vi "SWLDA.vi"(5 "premove":dbl=0.5, 7 "penter":dbl=0.4, 8 "Maximum_Iteration":dbl=88.0, 10 "ERP_NonTarget":path=path "C:/Users/Jaehong/Desktop/안전복지프로젝트/LabVIEW/RSVP_offline_onine/분석데이터/전선미_RSVP_Training_Test(LDA)/2014-08-29/ERP_Parameters_of_NonTarget_prior.txt", 11 "ERP_Target":path=path "C:/Users/Jaehong/Desktop/안전복지프로젝트/LabVIEW/RSVP_offline_onine/분석데이터/전선미_RSVP_Training_Test(LDA)/2014-08-29/ERP_Parameters_of_Target_prior.txt") -> (0 "in":dbl[](array[numeric]), 3 "Weight":dbl[](array[numeric]))   [LabVIEW 2014]
uses:
  <vilib>/Analysis/baseanly.llb/Vector x A.vi
  <vilib>/Utility/file.llb/Read From Spreadsheet File (DBL).vi
  <vilib>/Analysis/Matrix/Numeric/Conversions/Array To Matrix - RA.vi
  <vilib>/Analysis/NI_AALBase.lvlib
  <vilib>/Analysis/Matrix/NI_Matrix.lvlib
panel:
  out "biase":dbl[](array[numeric])
  out "Nontarget_mean":dbl[](array[numeric])
  out "Target_mean":dbl[](array[numeric])
  out "Label":dbl[](array[numeric])
  # "Target/Non-Target of MATLAB"
  # "var_argin part of MATLAB"
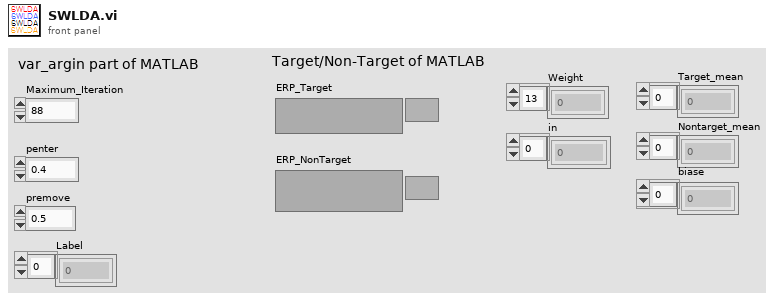
[diagram p1: front panel]
types:
  T1 = typedef "NI_Matrix.lvlib/RealMatrix.ctl" = dbl[][]
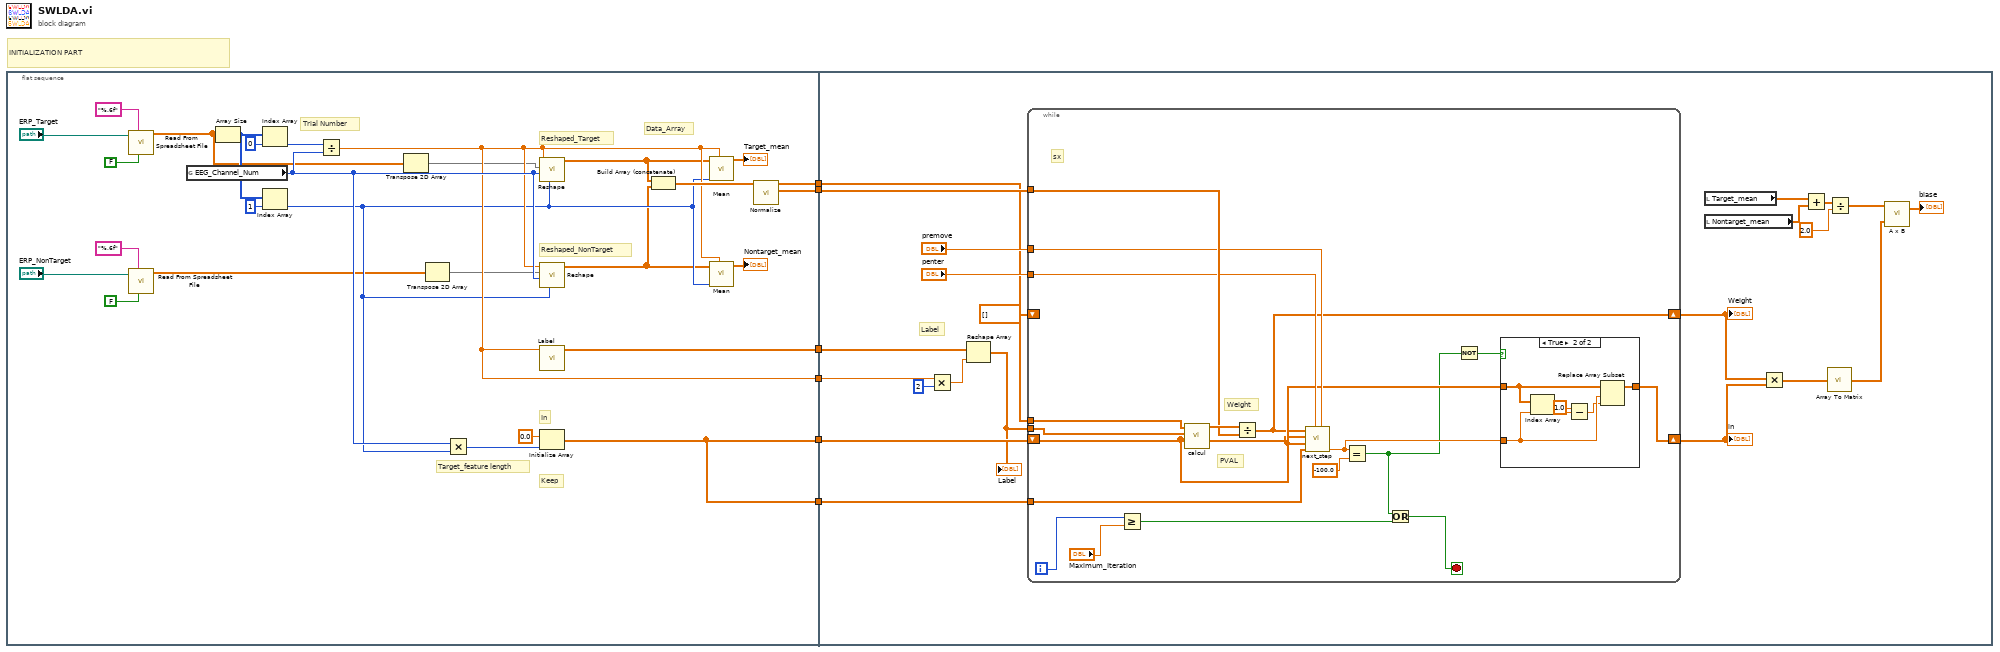
[diagram p0: block diagram]
diagram:
  # "INITIALIZATION PART"
  n1 = flat-sequence {
    tunnel: [w17] -> w6
    tunnel: [w17] -> w5
    tunnel: [w21] -> w4
    tunnel: [w20] -> w3
    tunnel: [w19] -> w2
    tunnel: [w15] -> w1
    tunnel: w6 -> [w55]
    tunnel: w5 -> [w50]
    tunnel: w4 -> [w56]
    tunnel: w3 -> [w46]
    tunnel: w2 -> [w53]
    tunnel: w1 -> [w45]
    frame #0 {
      # "Keep"
      # "In"
      # "Target_feature length"
      # "Data_Array"
      # "Reshaped_NonTarget"
      # "Reshaped_Target"
      # "Trial Number"
      n2 = call-poly <vilib>:"Read From Spreadsheet File.vi"("transpose (no:F)"=FALSE, "format (%.3f)"="%.6f", "file path (dialog if empty)"="ERP_Target") -> ("all rows"=w11:dbl[][])  [unwired: 4 in, 4 out]
      n3 = call-poly <vilib>:"Read From Spreadsheet File.vi"("transpose (no:F)"=FALSE, "format (%.3f)"="%.6f", "file path (dialog if empty)"="ERP_NonTarget") -> ("all rows"=w12:dbl[][])  [unwired: 4 in, 4 out]
      n4 = global read "Control_Panel.vi" "EEG_Channel_Num"() -> (w24:i32)
      n5 = Array Size(array=w11) -> (size(s)=w26:i32[])
      n6 = Index Array(array=w26, index=0) -> (element=w25:i32)
      n7 = Index Array(array=w26, index=1) -> (element=w14:i32)
      n8 = Divide(x=w25, y=w24) -> (x/y=w15:dbl)
      n9 = Transpose 2D Array(2D array=w11) -> (transposed array=w10:dbl[][])
      n10 = Transpose 2D Array(2D array=w12) -> (transposed array=w9:dbl[][])
      n11 = Multiply(x=w24, y=w14) -> (x*y=w23:i32)
      n12 = call "Reshape.vi"("Numeric"=w14, "EEG_Channel_Num"=w24, "all rows"=w10, "Numeric 2"=w15) -> ("Array"=w7:dbl[][])  [unwired: 7 in]
      n13 = call "Reshape.vi"("Numeric"=w14, "EEG_Channel_Num"=w24, "all rows"=w9, "Numeric 2"=w15) -> ("Array"=w8:dbl[][])  [unwired: 7 in]
      n14 = call "Label.vi"("Numeric"=w15) -> ("Array"=w21:dbl[][])  [unwired: 10 in]
      n15 = Initialize Array(0.0 ("element"), w23) -> (w17:dbl[])
      n16 = Build Array (concatenate)(w7, w8) -> (w18:dbl[][])
      n17 = call "Mean.vi"("trial_number"=w15, "feature_number"=w14, "Target/NonTarget"=w7) -> ("mean"=→"Target_mean":dbl[])  [unwired: 8 in]
      n18 = call "Mean.vi"("trial_number"=w15, "feature_number"=w14, "Target/NonTarget"=w8) -> ("mean"=→"Nontarget_mean":dbl[])  [unwired: 8 in]
      n19 = call "Normalize.vi"("Data"=w18) -> ("sx"=w19:dbl[], "Data_out"=w20:dbl[][])  [unwired: 8 in, 1 out]
    }
    frame #1 {
      # "Label"
      n20 = Multiply(x=w45, y=2) -> (x*y=w48:dbl)
      n21 = Reshape Array(w56, w48) -> (w54:dbl[])
      "Label" <- w54
      n22 = while {
        shift-right: [w62] -> w39
        shift-left: w55 -> [w63]
        tunnel: w54 -> [w71]
        tunnel: w46 -> [w70]
        tunnel: w53 -> [w68]
        tunnel: "penter" -> [w67]
        tunnel: "premove" -> [w66]
        tunnel: w50 -> [w65]
        shift-right: [w61] -> w40
        shift-left: dbl[] [] -> [_]
        i -> [w75]
        stop <- w72 stop-if-true
        # "sx"
        # "PVAL"
        # "Weight"
        n23 = Greater Or Equal?(x=w75, y="Maximum_Iteration") -> (x >= y?=w73:bool)
        n24 = call "calcul.vi"("In"=w63, "Label (y)"=w71, "Data (allx)"=w70) -> ("PVAL"=w57:dbl[], "B"=w69:dbl[])  [unwired: 7 in]
        n25 = Divide(x=w69, y=w68) -> (x/y=w61:dbl[])
        n26 = call "next_step.vi"("premove"=w66, "penter"=w67, "keep"=w65, "in"=w63, "PVal"=w57, "B"=w61) -> ("swap"=w60:dbl)  [unwired: 4 in, 1 out]
        n27 = Equal?(x=w60, y=-100.0) -> (x = y?=w58:bool)
        n28 = Or(x=w58, y=w73) -> (x .or. y?=w72:bool)
        n29 = Not(x=w58) -> (.not. x?=w59:bool)
        n30 = case shown="True" w59 {
          tunnel: w63 -> [w76 w81]
          tunnel: w60 -> [_ w80]
          tunnel: [w76 w82] -> w62
          frame False {
          }
          frame True {
            n31 = Index Array(array=w81, index=w80) -> (element=w79:dbl)
            n32 = Subtract(x=1.0, y=w79) -> (x-y=w77:dbl)
            n33 = Replace Array Subset(array=w81, new element=w77, index=w80) -> (w82:dbl[])
          }
        }
      }
      "Weight" <- w40
      "in" <- w39
      n34 = local read "Target_mean"() -> (w44:dbl[])
      n35 = local read "Nontarget_mean"() -> (w43:dbl[])
      n36 = Multiply(x=w40, y=w39) -> (x*y=w37:dbl[])
      n37 = Add(x=w44, y=w43) -> (x+y=w42:dbl[])
      n38 = call-poly <vilib>:"Array To Matrix.vi"("Real 1D Array"=w37) -> ("Real Matrix (Column Vector)"=w36:T1)
      n39 = Divide(x=w42, y=2.0) -> (x/y=w38:dbl[])
      n40 = call-poly <vilib>:"A x B.vi"("Matrix A"=w36, "Vector V'"=w38) -> ("V' x A"=→"biase":dbl[])  [unwired: 1 out]
    }
  }
